vi "create default channels.vi"() -> (0 "error out":errorcluster, 1 "names":string[](array[string]), 2 "channels":refnum<class "TBM channel.lvclass">[](array[class]), 3 "module":refnum<class "tag bus configurable plugin module configuration.lvclass">, 5 "instance identifier":string)   [LabVIEW 2013, in "io plugin tests.lvlib"]
uses:
  io plugin tests.lvlib
  <vilib>/NI/Tag Bus Module Framework/channel/TBM channel.lvclass
  module/configuration/tag bus configurable plugin module configuration.lvclass
  <vilib>/NI/Tag Bus Module Framework/channel/channel classification.ctl
  <vilib>/NI/Tag Bus Module Framework/root configuration/TBM configuration.lvclass
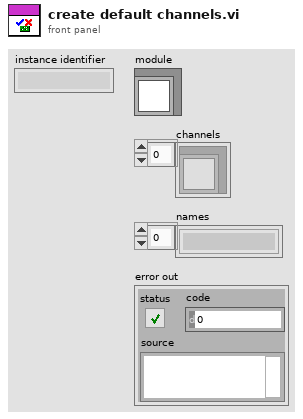
[diagram p1: front panel]
types:
  T1 = typedef "TBM channel.lvclass/channel classification.ctl" = enum16{"input data", "output data", "processing parameter", "processing result"}
  T2 = typedef "tag bus.lvlib/tag descriptor.lvclass/Data Type.ctl" = enum16{"Double", "Single", "I64", "I32", "I16", "I8", "U64", "U32", "U16", "U8", "Boolean", "String", "Array of Double", "Array of Single", "Array of I64", "Array of I32", "Array of I16", "Array of I8", "Array of U64", "Array of U32", "Array of U16", "Array of U8", "Array of Boolean", "Array of String"}
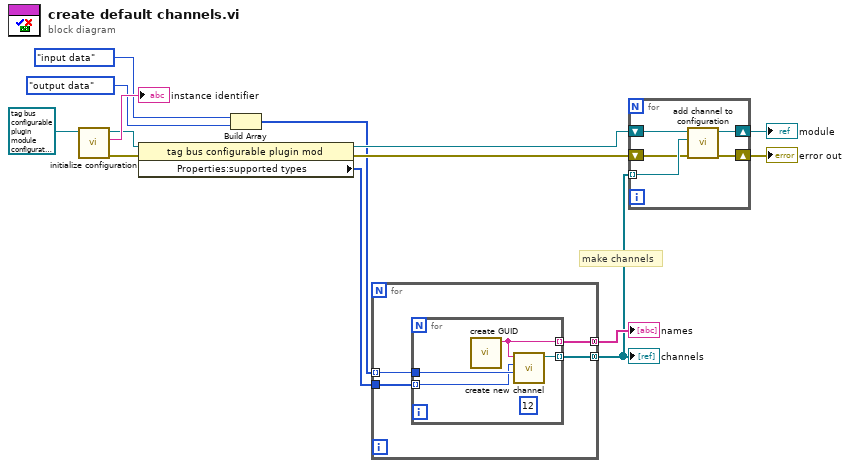
[diagram p0: block diagram]
diagram:
  # "make channels"
  n1 = call-dynamic "initialize configuration.vi"("configuration in"=refnum<class "tag bus configurable plugin module configuration.lvclass"> refnum ("tag bus configurable plugin module configuration")) -> ("error out"=w12:errorcluster, "instance identifier"=→"instance identifier":string, "configuration out"=w9:refnum<class "tag bus configurable plugin module configuration.lvclass">)  [unwired: 8 in]
  n2 = property class="tag bus configurable plugin mod"(reference=w9, error in=w12) -> (reference out=w4:refnum<class "tag bus configurable plugin module configuration.lvclass">, error out=w11:errorcluster, "Properties:supported types"=w5:T2[])
  n3 = Build Array(channel_classification."input data" ("channel classification"), channel_classification."output data" ("channel classification")) -> (w3:T1[])
  n4 = for {
    tunnel: w3 -> [w18] mode=indexing
    tunnel: [w16] -> w8 mode=concatenating
    tunnel: w5 -> [w17]
    tunnel: [w15] -> w10 mode=concatenating
    n5 = for {
      tunnel: w18 -> [w21]
      tunnel: [w22] -> w16 mode=indexing
      tunnel: w17 -> [w20] mode=indexing
      tunnel: [w19] -> w15 mode=indexing
      (unwired) 12
      n6 = call <vilib>:"create GUID.vi"() -> ("uuid"=w19:string)  [unwired: 11 in]
      n7 = call <vilib>:"create new channel.vi"("channel classification"=w21, "data type"=w20, "channel name"=w19) -> ("channel"=w22:refnum<class "TBM channel.lvclass">)  [unwired: 8 in]
    }
  }
  "names" <- w10
  "channels" <- w8
  n8 = for {
    tunnel: w8 -> [w25] mode=indexing
    shift-right: [w26] -> w7
    shift-left: w4 -> [w27]
    shift-right: [w23] -> w14
    shift-left: w11 -> [w24]
    n9 = call "add channel to configuration.vi"("error in"=w24, "channel"=w25, "tag bus configurable plugin module configuration in"=w27) -> ("error out"=w23:errorcluster, "tag bus configurable plugin module configuration out"=w26:refnum<class "tag bus configurable plugin module configuration.lvclass">)  [unwired: 7 in]
  }
  "error out" <- w14
  "module" <- w7
